vi "Init.vi"(8 "error in (no error)":errorcluster, 11 "Data in":refnum<class "Event_Bus.lvclass">) -> (0 "error out":errorcluster, 3 "Data out":refnum<class "Event_Bus.lvclass">)   [LabVIEW 2021, in "Event_Bus.lvclass"]
doc: "Abstract Data Classes 2.1.1.12\nTim Streeter - TSA\nCopyright (c) 2024, TSA"
uses:
  Event_Bus.lvclass
  C:/Users/timst/Documents/Repositories/Omni-Bus/Source/Omni-Bus/Bus Access/Bus_Access.lvclass
  Event_Bus.lvclass/Event_Bus.ctl
  Omni-Bus/Bus Access/Bus_Access.lvclass/Bus_Access.ctl
  <vilib>/TSA/Abstract Data Classes/Abs_Types/Value/Abs_Value.lvclass
  <vilib>/TSA/Abstract Data Classes/Abs_Types/Boolean/Abs_Boolean.lvclass
  Support/Event Type/OnChange/Bool/OnChange_Boolean.lvclass
  C:/Users/timst/Documents/Repositories/Omni-Bus/Source/Event Bus/Support/Event_Polled Type.lvclass
  C:/Program Files (x86)/National Instruments/LabVIEW 2021/vi.lib/TSA/Abstract Data Classes/Abs_Types/Type/Abs_Type.lvclass
  Support/Event Type/OnChange/Bool/OnChange_Boolean.lvclass/OnChange_Boolean.ctl
  Support/Event Source/Event_Source.lvclass/Event_Source.ctl
  Support/Event Type/OnChange/Bool/Properties/Write Data Type.vi
  Omni-Bus/Bus Access/Properties/Read Values.vi
  Omni-Bus/Bus Access/Properties/Read Tags.vi
  Properties/Read Buses.vi
  Properties/Read Tags to Event.vi
  Omni-Bus/Bus Access/Properties/Read Tag Root.vi
  Properties/Write Event_Source.vi
  Omni-Bus/Bus Access/Properties/Write Values.vi
  Omni-Bus/Bus Access/Properties/Write Tags.vi
  Properties/Read Event_Source.vi
  Support/Event Source/Properties/Write Events.vi
  Omni-Bus/Bus Access/Bus_Access.lvclass
  <vilib>/TSA/Abstract Data Classes/Abs_Types/Type/Abs_Type.lvclass
  Support/Event Source/Event_Source.lvclass
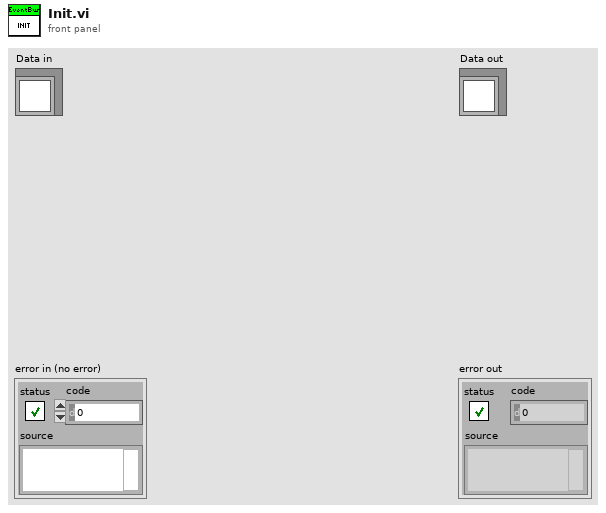
[diagram p1: front panel]
types:
  T1 = typedef "NI_Data Type.lvlib/Data Type.ctl" = enum8{"Invalid Type", "Void", "I8", "I16", "I32", "I64", "U8", "U16", "U32", "U64", "Single Float", "Double Float", "Extended Float", "Single Complex", "Double Complex", "Extended Complex", "Enum U8", "Enum U16", "Enum U32", "Enum U64", "Single Float With Unit", "Double Float With Unit", "Extended Float With Unit", "Single Complex with Unit", "Double Complex with Unit", "Extended Complex with Unit", "Boolean", "String", "Path", "Picture", "Tag", "Array", "Cluster", "Variant", "LV Variant", "Waveform", "Timestamp", "Digital Waveform", "Digital Data", "ExpressData", "Refnum", "External Data", "VI", "Poly VI", "LabVIEW Class Instance", "Fixed Point", "Set Collection", "Map Collection"}
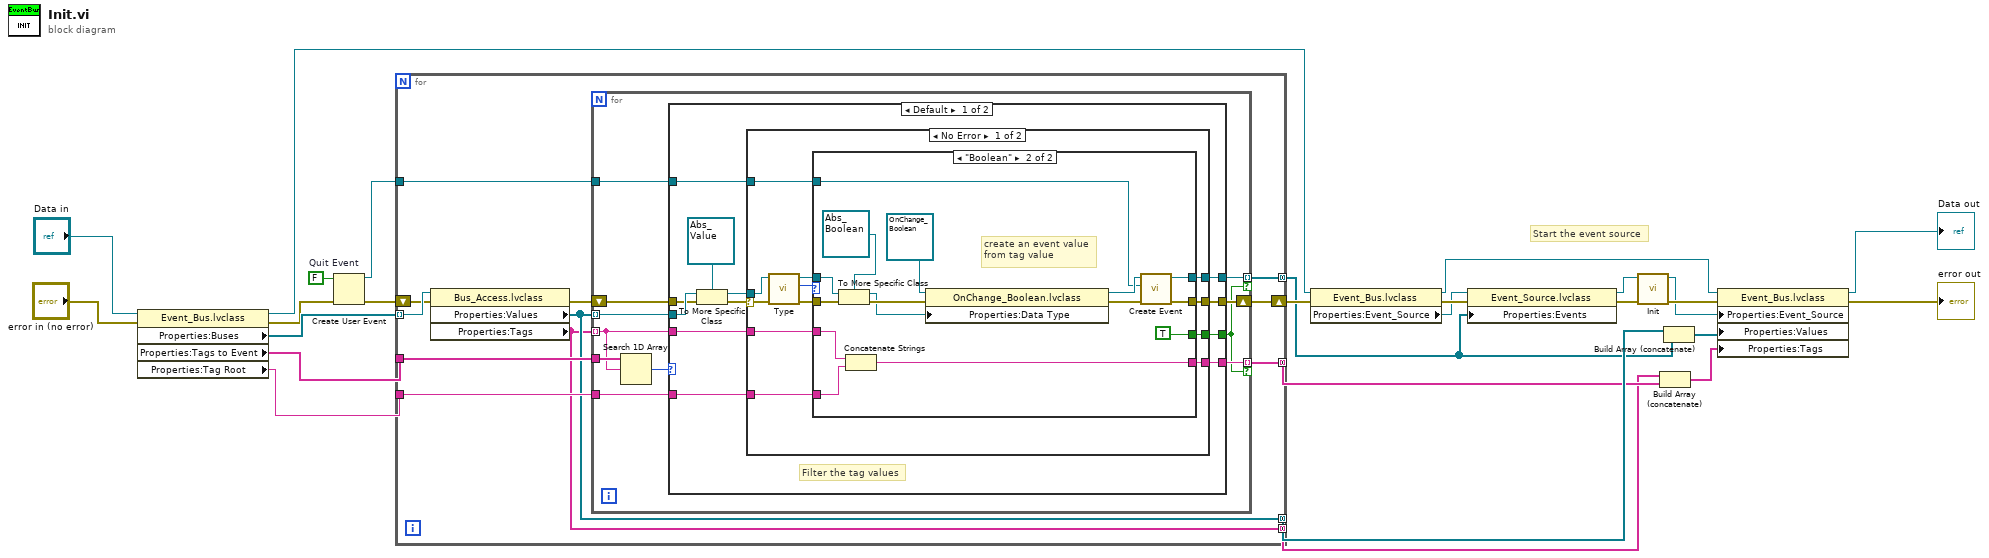
[diagram p0: block diagram]
diagram:
  w4 = FALSE  # Quit Event
  # "Start the event source"
  n1 = property class="Event_Bus.lvclass"(reference="Data in", error in="error in (no error)") -> (reference out=w11:refnum<class "Event_Bus.lvclass">, error out=w3:errorcluster, "Properties:Buses"=w24:refnum<class "Bus_Access.lvclass">[], "Properties:Tags to Event"=w21:string[], "Properties:Tag Root"=w20:string)
  n2 = Create User Event(user event datatype=w4, error in=w3) -> (user event=w1:refnum<user-event>, error out=w2:errorcluster)
  n3 = for {
    tunnel: w24 -> [w37] mode=indexing
    shift-right: [w33] -> w12
    shift-left: w2 -> [w36]
    tunnel: w21 -> [w35]
    tunnel: w20 -> [w32]
    tunnel: [w29] -> w17 mode=concatenating
    tunnel: [w31] -> w5 mode=concatenating
    tunnel: [w30] -> w19 mode=concatenating
    tunnel: [w28] -> w16 mode=concatenating
    tunnel: w1 -> [w27]
    n4 = property class="Bus_Access.lvclass"(reference=w37, error in=w36) -> (error out=w34:errorcluster, "Properties:Values"=w30:refnum<class "Abs_Type.lvclass">[], "Properties:Tags"=w28:string[])  [unwired: 1 out]
    n5 = for {
      tunnel: w30 -> [w46] mode=indexing
      tunnel: w28 -> [w42] mode=indexing
      tunnel: w35 -> [w48]
      shift-right: [w44] -> w33
      shift-left: w34 -> [w45]
      tunnel: [w43] -> w31 mode=indexing if=w39
      tunnel: w32 -> [w41]
      tunnel: [w40] -> w29 mode=indexing if=w39
      tunnel: w27 -> [w38]
      n6 = Search 1D Array(1D array=w48, element=w42) -> (index of element=w47:i32)  [unwired: 1 in]
      n7 = case shown="Default" w47 {
        tunnel: w46 -> [w60 _]
        tunnel: w45 -> [w59 w90]
        tunnel: [w55 w90] -> w44
        tunnel: [w54 _] -> w43
        tunnel: w42 -> [w53 _]
        tunnel: w41 -> [w52 _]
        tunnel: [w51 _] -> w40
        tunnel: [w50 _] -> w39
        tunnel: w38 -> [w49 _]
        frame Default {
          # "Filter the tag values"
          n8 = To More Specific Class(target class=refnum<class "Abs_Value.lvclass"> refnum ("Abs_Value.lvclass"), reference=w60, error in=w59) -> (specific class reference=w56:refnum<class "Abs_Value.lvclass">, error out=w57:errorcluster)
          n9 = case shown="No Error" w57 {
            selector: w57 -> [w72 w89]
            tunnel: w56 -> [w71 _]
            tunnel: [w67 w89] -> w55
            tunnel: [w66 _] -> w54
            tunnel: w53 -> [w65 _]
            tunnel: w52 -> [w64 _]
            tunnel: [w63 _] -> w51
            tunnel: [w62 _] -> w50
            tunnel: w49 -> [w61 _]
            frame No Error {
              n10 = call-dynamic "Type.vi"("error in (no error)"=w72, "Element in"=w71) -> ("error out"=w69:errorcluster, "Type"=w70:T1, "Element out"=w68:refnum<class "Abs_Value.lvclass">)  [unwired: 7 in]
              n11 = case shown="\"Boolean\"" w70 {
                tunnel: w69 -> [w73 w87]
                tunnel: w68 -> [_ w86]
                tunnel: [w73 w77] -> w67
                tunnel: [_ w75] -> w66
                tunnel: w65 -> [_ w82]
                tunnel: w64 -> [_ w81]
                tunnel: [_ w80] -> w63
                tunnel: [_ TRUE] -> w62
                tunnel: w61 -> [_ w74]
                frame Default {
                }
                frame "Boolean" {
                  # "create an event value\nfrom tag value"
                  n12 = To More Specific Class(target class=refnum<class "Abs_Boolean.lvclass"> refnum ("Data Type"), reference=w86, error in=w87) -> (specific class reference=w83:refnum<class "Abs_Boolean.lvclass">, error out=w84:errorcluster)
                  n13 = Concatenate Strings(w82, w81) -> (w80:string)
                  n14 = property class="OnChange_Boolean.lvclass"(reference=refnum<class "OnChange_Boolean.lvclass"> refnum ("OnChange_Boolean.lvclass"), error in=w84, "Properties:Data Type"=w83) -> (reference out=w76:refnum<class "OnChange_Boolean.lvclass">, error out=w78:errorcluster)
                  n15 = call-dynamic "Create Event.vi"("error in (no error)"=w78, "Quit Event"=w74, "OnChange_Boolean in"=w76) -> ("error out"=w77:errorcluster, "OnChange_Boolean out"=w75:refnum<class "OnChange_Boolean.lvclass">)  [unwired: 7 in]
                }
              }
            }
            frame Error {
            }
          }
        }
        frame -1 {
        }
      }
    }
  }
  n16 = property class="Event_Bus.lvclass"(reference=w11, error in=w12) -> (reference out=w10:refnum<class "Event_Bus.lvclass">, error out=w9:errorcluster, "Properties:Event_Source"=w8:refnum<class "Event_Source.lvclass">)
  n17 = property class="Event_Source.lvclass"(reference=w8, error in=w9, "Properties:Events"=w5) -> (reference out=w6:refnum<class "Event_Source.lvclass">, error out=w7:errorcluster)
  n18 = call-dynamic "Init.vi"("error in (no error)"=w7, "Data in"=w6) -> ("error out"=w14:errorcluster, "Data out"=w13:refnum<class "Event_Source.lvclass">)  [unwired: 8 in]
  n19 = Build Array (concatenate)(w16, w17) -> (w15:string[])
  n20 = Build Array (concatenate)(w19, w5) -> (w18:refnum<class "Abs_Type.lvclass">[])
  n21 = property class="Event_Bus.lvclass"(reference=w10, error in=w14, "Properties:Event_Source"=w13, "Properties:Values"=w18, "Properties:Tags"=w15) -> (reference out=→"Data out":refnum<class "Event_Bus.lvclass">, error out=→"error out":errorcluster)
